vi "Change Desired Temperature.vi"(8 "error in (no error)":errorcluster caption="entrée d'erreur (pas d'erreur)", 10 "Desired Temperature":dbl, 11 "Cooler UI with Events en entrée":refnum<class "Cooler UI with Events.lvclass">) -> (0 "error out":errorcluster caption="sortie d'erreur", 3 "Cooler UI with Events en sortie":refnum<class "Cooler UI with Events.lvclass">)   [LabVIEW 2015, in "Cooler UI.lvlib" / "Cooler UI with Events.lvclass"]
uses:
  Cooler UI with Events.lvclass
  Cooler UI with Events.lvclass/Cooler UI with Events.ctl
  Level Controller/Level Controller Messages/Write Deadband Msg/Write Deadband Msg.lvclass/Write Deadband Msg.ctl
  <vilib>/ActorFramework/Message Enqueuer/Message Enqueuer.lvclass/Message Enqueuer.ctl
  <vilib>/ActorFramework/Message Enqueuer/Enqueue.vi
  <vilib>/ActorFramework/Message Priority Queue/Priority Enqueue.vi
  Level Controller/Level Controller Messages/Write Deadband Msg/Write Deadband Msg.lvclass
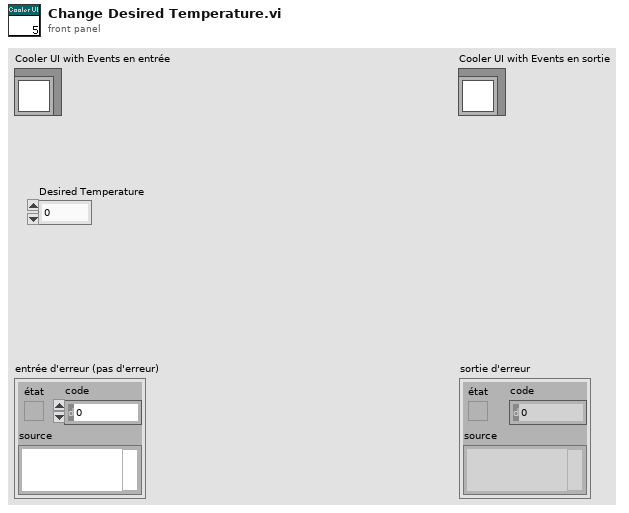
[diagram p1: front panel]
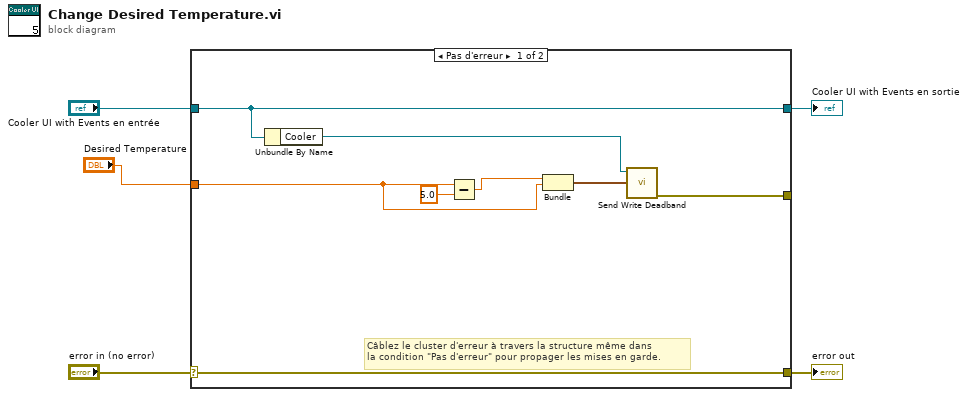
[diagram p0: block diagram]
diagram:
  n1 = case shown="Pas d'erreur" "error in (no error)" {
    selector: "error in (no error)" -> [w13 w15]
    tunnel: [w13 w15] -> w4
    tunnel: [w7 w14] -> w2
    tunnel: "Cooler UI with Events en entrée" -> [w7 w14]
    tunnel: "Desired Temperature" -> [w10 _]
    tunnel: [w8 _] -> _
    frame No Error {
      # "Câblez le cluster d'erreur à travers la structure même dans\nla condition \"Pas d'erreur\" pour propager les mises en garde."
      n2 = Unbundle By Name(w7) -> ("Cooler"=w6:refnum<class "Message Enqueuer.lvclass">)
      n3 = Subtract(x=w10, y=5.0) -> (x-y=w11:dbl)
      n4 = Bundle(w11, "Desired Temperature"=w10) -> (w9:cluster{dbl, "Desired Temperature":dbl})  [unwired: 1 in]
      n5 = call "Send Write Deadband.vi"("Deadband"=w9, "Message Enqueuer"=w6) -> ("error out"=w8:errorcluster)  [unwired: 8 in, 1 out]
    }
    frame Error {
    }
  }
  "error out" <- w4
  "Cooler UI with Events en sortie" <- w2
